vi "Parse GET Object Result.vi"(8 "error in (no error)":errorcluster, 11 "Response header":string) -> (0 "error out":errorcluster, 3 "GetObjectResult":T1)   [LabVIEW 2015, in "NI_AWS_S3.lvlib" / "Object.lvclass"]
uses:
  Object.lvclass
  GET Object Result Parameters.ctl
  NI_AWS_S3.lvlib
  Core/NI_AWS_Core.lvlib
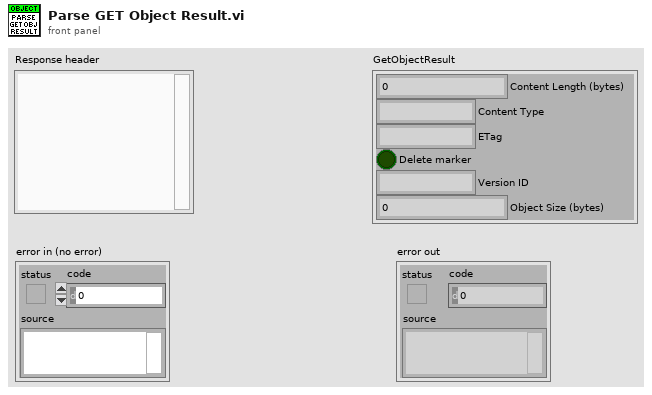
[diagram p1: front panel]
types:
  T1 = typedef "NI_AWS_S3.lvlib/GET Object Result Parameters.ctl" = cluster{"Content Length (bytes)":u64, "Content Type":string, "ETag":string, "Delete marker":bool, "Version ID":string, "Object Size (bytes)":u64}
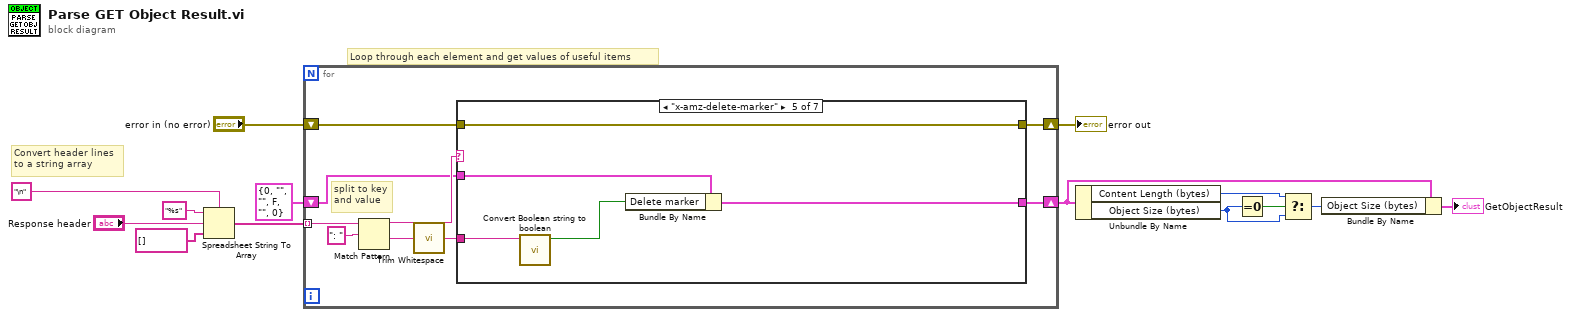
[diagram p0: block diagram]
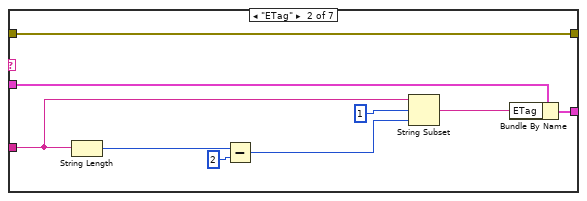
[diagram p3: hidden frame]
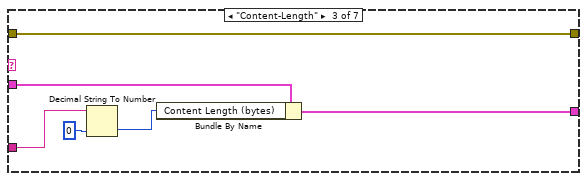
[diagram p4: hidden frame]
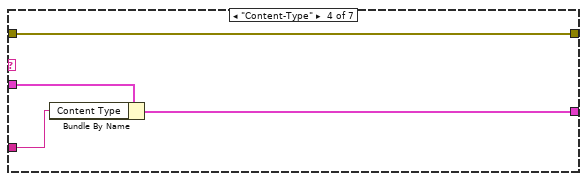
[diagram p5: hidden frame]
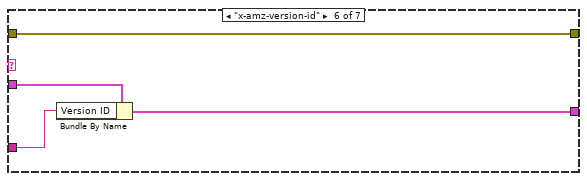
[diagram p6: hidden frame]
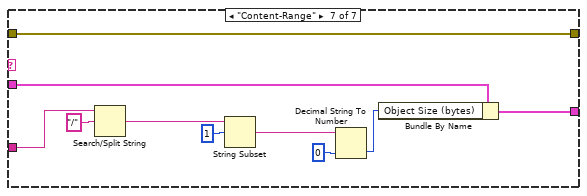
[diagram p7: hidden frame]
diagram:
  # "Loop through each element and get values of useful items"
  # "Convert header lines\nto a string array"
  n1 = Spreadsheet String To Array(delimiter (Tab)="\n", format string="%s", spreadsheet string="Response header", array type (2D Dbl)=string[] []) -> (array=w11:string[])
  n2 = for {
    tunnel: w11 -> [w23] mode=indexing
    shift-right: [w19] -> w7
    shift-left: "error in (no error)" -> [w20]
    shift-right: [w17] -> w3
    shift-left: T1 {"Content Length (bytes)"=0, "Content Type"="", "ETag"="", "Delete marker"=FALSE, "Version ID"="", "Object Size (bytes)"=0} ("GetObjectResult") -> [w18]
    # "split to key\nand value"
    n3 = Match Pattern(string=w23, regular expression=": ") -> (before substring=w21:string, after substring=w16:string)  [unwired: 1 in, 2 out]
    n4 = call <vilib>:"Trim Whitespace.vi"("string"=w16) -> ("trimmed string"=w15:string)  [unwired: 1 in]
    n5 = case shown="\"x-amz-delete-marker\"" w21 {
      tunnel: [w25 w34 w35 w41 w47 w51 w59] -> w19
      tunnel: w20 -> [w25 w34 w35 w41 w47 w51 w59]
      tunnel: w15 -> [_ w32 w40 w43 w46 w50 w58]
      tunnel: w18 -> [w24 w28 w38 w44 w49 w53 w57]
      tunnel: [w24 w26 w36 w42 w48 w52 w56] -> w17
      frame Default {
      }
      frame "ETag" {
        n6 = String Length(string=w32) -> (length=w31:i32)
        n7 = Subtract(x=w31, y=2) -> (x-y=w30:i32)
        n8 = String Subset(string=w32, offset (0)=1, length (rest)=w30) -> (substring=w27:string)
        n9 = Bundle By Name(cluster=w28, "ETag"=w27) -> (w26:T1)
      }
      frame "Content-Length" {
        n10 = Decimal String To Number(string=w40, default (0L)=u64 0 ("default (0 I32)")) -> (number=w37:u64)  [unwired: 1 in, 1 out]
        n11 = Bundle By Name(cluster=w38, "Content Length (bytes)"=w37) -> (w36:T1)
      }
      frame "Content-Type" {
        n12 = Bundle By Name(cluster=w44, "Content Type"=w43) -> (w42:T1)
      }
      frame "x-amz-delete-marker" {
        n13 = call "Convert Boolean string to boolean.vi"("Boolean String"=w46) -> ("Boolean"=w45:bool)  [unwired: 10 in]
        n14 = Bundle By Name(cluster=w49, "Delete marker"=w45) -> (w48:T1)
      }
      frame "x-amz-version-id" {
        n15 = Bundle By Name(cluster=w53, "Version ID"=w50) -> (w52:T1)
      }
      frame "Content-Range" {
        n16 = Search/Split String(string=w58, search string/char (-)="/") -> (match + rest of string=w62:string)  [unwired: 1 in, 2 out]
        n17 = String Subset(string=w62, offset (0)=1) -> (substring=w60:string)  [unwired: 1 in]
        n18 = Decimal String To Number(string=w60, default (0L)=u64 0) -> (number=w55:u64)  [unwired: 1 in, 1 out]
        n19 = Bundle By Name(cluster=w57, "Object Size (bytes)"=w55) -> (w56:T1)
      }
    }
  }
  "error out" <- w7
  n20 = Unbundle By Name(w3) -> ("Content Length (bytes)"=w5:u64, "Object Size (bytes)"=w4:u64)
  n21 = Equal To 0?(x=w4) -> (x = 0?=w6:bool)
  n22 = Select(t=w5, s=w6, f=w4) -> (s? t:f=w2:u64)
  n23 = Bundle By Name(cluster=w3, "Object Size (bytes)"=w2) -> (→"GetObjectResult":T1)
